vi "Camera Set.vi"(0 "Camera Data":T1) -> ()   [LabVIEW 2012]
uses:
  BotStatus.vi
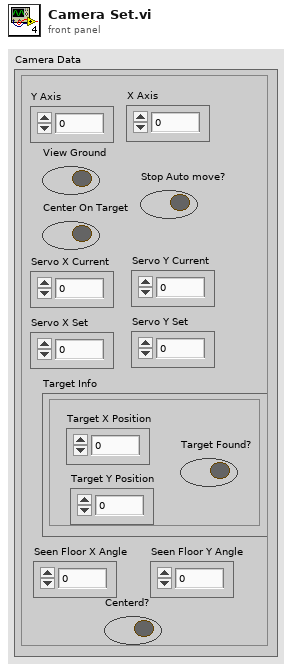
[diagram p1: front panel]
types:
  T1 = cluster{"Y Axis":dbl, "X Axis":dbl, "View Ground":bool, "Center On Target":bool, "Stop Auto move?":bool, "Servo X Current":dbl, "Servo Y Current":dbl, "Target Info":cluster{"Target Found?":bool, "Target X Position":dbl, "Target Y Position":dbl}, "Seen Floor X Angle":dbl, "Seen Floor Y Angle":dbl, "Centerd?":bool, "Servo X Set":dbl, "Servo Y Set":dbl}
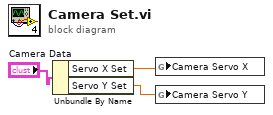
[diagram p0: block diagram]
diagram:
  n1 = Unbundle By Name("Camera Data") -> ("Servo X Set"=w2:dbl, "Servo Y Set"=w1:dbl)
  n2 = global write "BotStatus.vi" "Camera Servo X"(w2) -> ()
  n3 = global write "BotStatus.vi" "Camera Servo Y"(w1) -> ()
